vi "添加启动项.vi"(8 "error in (no error)":errorcluster caption="错误输入（无错误）", 11 "启动文件路径":path) -> (0 "error out":errorcluster caption="错误输出", 3 "添加成功标记":bool)   [LabVIEW 2016, in "数据传输系统-04.lvlib"]
uses:
  <vilib>/registry/registry.llb/Registry RtKey.ctl
  <vilib>/registry/registry.llb/Write Registry Value Simple STR.vi
panel:
  out "结果字符串":string
  out "字符串":string
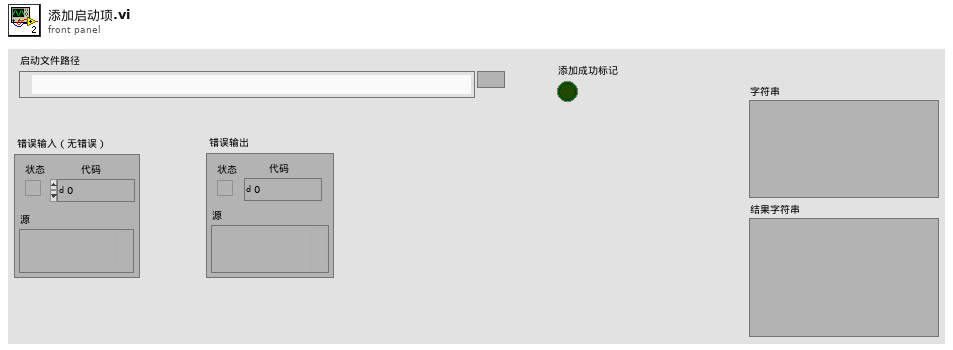
[diagram p1: front panel]
types:
  T1 = typedef "Registry RtKey.ctl" = enum32{"HKEY_CLASSES_ROOT", "HKEY_CURRENT_USER", "HKEY_LOCAL_MACHINE", "HKEY_USERS", "HKEY_PERFORMANCE_DATA", "HKEY_CURRENT_CONFIG", "HKEY_DYN_DATA"}
  T2 = typedef "Registry refnum.ctl" = refnum<k1>
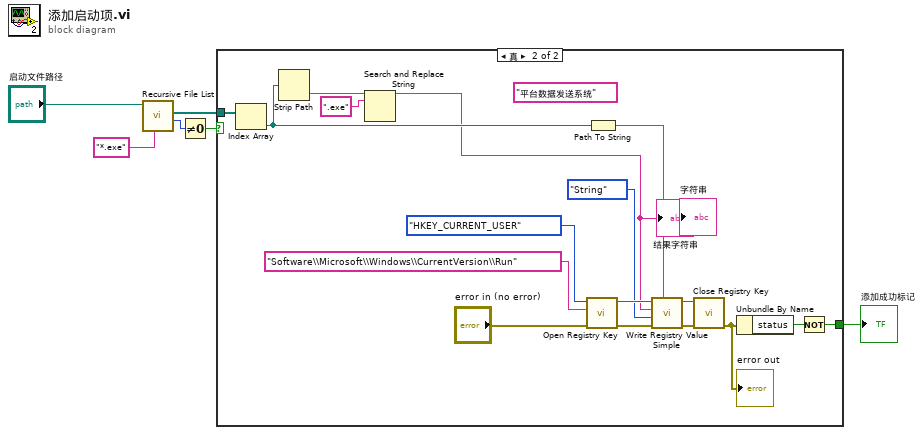
[diagram p0: block diagram]
diagram:
  n1 = call <vilib>:"Recursive File List.vi"("pattern"="*.exe", "Folder Path"="启动文件路径") -> ("Number of Files"=w3:i32, "All Files in Dir"=w4:path[])  [unwired: 5 in, 3 out]
  n2 = Not Equal To 0?(x=w3) -> (x != 0?=w2:bool)
  n3 = case shown="真" w2 {
    tunnel: w4 -> [_ w23]
    tunnel: [_ w9] -> w1
    frame False {
    }
    frame True {
      (unwired) "平台数据发送系统" ("value")
      n4 = Index Array(array=w23) -> (element=w22:path)  [unwired: 1 in]
      n5 = Strip Path(path=w22) -> (name=w21:string)  [unwired: 1 out]
      n6 = Search and Replace String(input string=w21, search string=".exe" ("搜索字符串")) -> (result string=w7:string)  [unwired: 6 in, 3 out]
      "结果字符串" <- w7
      n7 = call <vilib>:"Open Registry Key.vi"("error in (no error)"="error in (no error)", "subkey"="Software\\Microsoft\\Windows\\CurrentVersion\\Run", "root key (HKEY_LOCAL_MACHINE)"=Registry_RtKey."HKEY_CURRENT_USER") -> ("error out"=w17:errorcluster, "refnum out"=w16:T2)  [unwired: 7 in]
      n8 = Path To String(path=w22) -> (string=w8:string)
      "字符串" <- w8
      n9 = call-poly <vilib>:"Write Registry Value Simple.vi"("String/Binary data"=w8, "error in (no error)"=w17, "simple data type"=enum16{"String", "Binary", "DWORD"}."String", "value"=w7, "refnum"=w16) -> ("error out"=w19:errorcluster, "refnum out"=w18:T2)  [unwired: 3 in]
      n10 = call <vilib>:"Close Registry Key.vi"("error in (no error)"=w19, "refnum"=w18) -> ("error out"=w11:errorcluster)  [unwired: 5 in]
      "error out" <- w11
      n11 = Unbundle By Name(w11) -> ("status"=w10:bool)
      n12 = Not(x=w10) -> (.not. x?=w9:bool)
    }
  }
  "添加成功标记" <- w1
